vi "Galil_programDownload.vi"() -> ()   [LabVIEW 2011]
panel:
  in  "Galil.IGalil":refnum<k7>
  out "Library Version:":string
  out "Uploaded Program:":string
  out "error out":errorcluster
  out "Connected To:":string
  in  "Connection String:":string
  # "This vi Shows how to use the programDownload function of the Galil Communications Library.  \n\nIf Connection String is left blank, the vi will open the connections dialog when run.  If a value is input into Connection String, the vi will attempt to connect to the controller at that address (ie COM1 19200).\n\nThe vi downloads a porgram to the controller with the programDownload function.  It then uploads the program from the controller with the programUpload function and shows it on the front Panel"
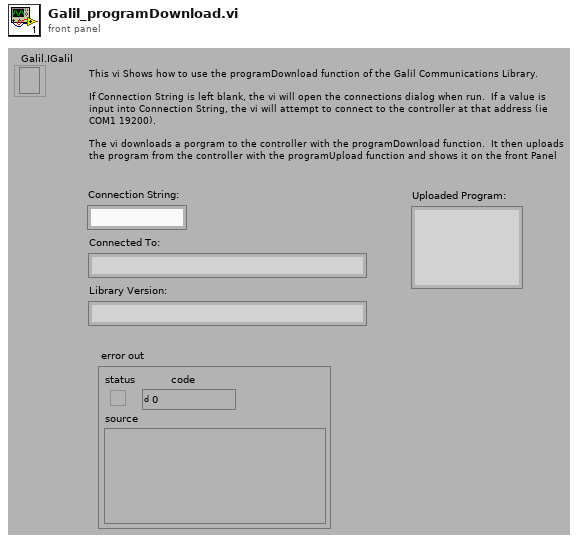
[diagram p1: front panel]
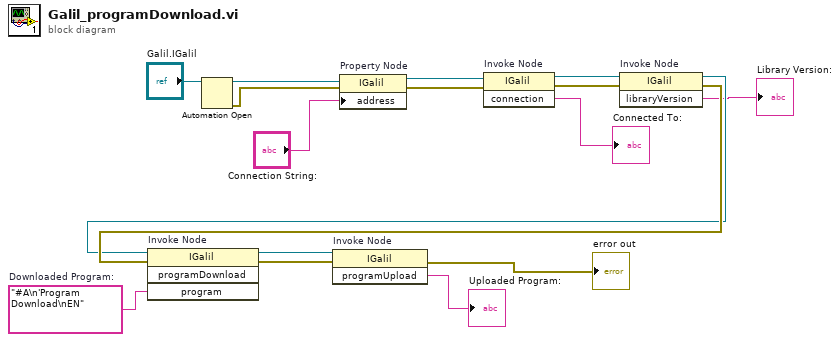
[diagram p0: block diagram]
diagram:
  w11 = "#A\n'Program Download\nEN"  # Downloaded Program:
  n1 = Automation Open(Automation Refnum="Galil.IGalil") -> (Automation Refnum=w17:refnum<k7>, error out=w15:errorcluster)  [unwired: 1 in, 2 out]
  n2 = property on="Property Node" class="IGalil"(reference=w17, error in=w15, "address"="Connection String:") -> (reference out=w16:refnum<k7>, error out=w14:errorcluster)
  n3 = invoke on="Invoke Node" class="IGalil" method="connection"(reference=w16, error in=w14) -> (reference out=w6:refnum<k7>, error out=w5:errorcluster, "connection"=→"Connected To:":string)  [unwired: 1 in]
  n4 = invoke on="Invoke Node" class="IGalil" method="libraryVersion"(reference=w6, error in=w5) -> (reference out=w3:refnum<k7>, error out=w4:errorcluster, "libraryVersion"=→"Library Version:":string)  [unwired: 1 in]
  n5 = invoke on="Invoke Node" class="IGalil" method="programDownload"(reference=w3, error in=w4, "program"=w11) -> (reference out=w10:refnum<k7>, error out=w9:errorcluster)  [unwired: 1 in, 2 out]
  n6 = invoke on="Invoke Node" class="IGalil" method="programUpload"(reference=w10, error in=w9) -> (error out=→"error out":errorcluster, "programUpload"=→"Uploaded Program:":string)  [unwired: 1 in, 1 out]
